vi "Heartbeat.vi"(7 "LabVIEW Web Service Request":refnum<class "Web Request.lvclass">, 11 "ClientName":string) -> ()   [LabVIEW 2017]
uses:
  <vilib>/wsapi/Web Request.lvclass
  ServerLib/SubLibs/WebServiceCommunication/WebServiceFGVcommands.ctl
  ServerLib/SubLibs/WebServiceCommunication/WebServiceCommunication.lvlib
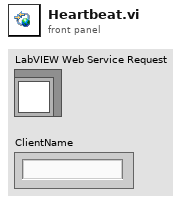
[diagram p1: front panel]
types:
  T1 = typedef "Server.lvlib/WebServiceCommunication.lvlib/WebServiceFGVcommands.ctl" = enum16{"Init", "Reset", "Heartbeat", "GetSRs", "SetSRs", "CheckClients", "GetClients"}
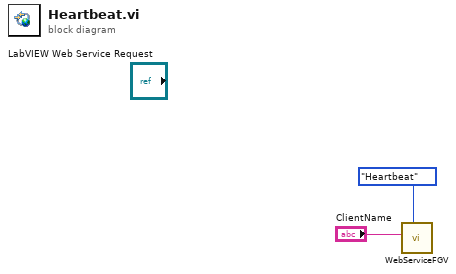
[diagram p0: block diagram]
diagram:
  n1 = call "WebServiceFGV.vi"("CMD"=WebServiceFGVcommands."Heartbeat", "ClientName"="ClientName") -> ()  [unwired: 7 in, 3 out]
